vi "Init.vi"() -> (3 "Auto Iterate Msg Strategy out":refnum<class "Auto Iterate Msg Strategy.lvclass">)   [LabVIEW 2021, in "Hello World Event.lvlib" / "Auto Iterate Msg Strategy.lvlib" / "Auto Iterate Msg Strategy.lvclass"]
uses:
  Auto Iterate Msg Strategy.lvclass
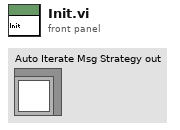
[diagram p1: front panel]
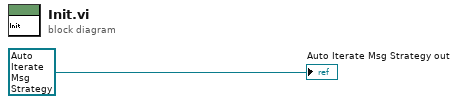
[diagram p0: block diagram]
diagram:
  "Auto Iterate Msg Strategy out" <- refnum<class "Auto Iterate Msg Strategy.lvclass"> refnum ("TEMPLATE Msg Strategy out")
